vi "Convert Sample Rate MHz to and from Enum.vi"(10 "Sample Frequency enum in":T1=enum."100MHz", 11 "MHz in":u8) -> (2 "MHz out":u8, 3 "Sample Frequency enum out":T1=enum."200MHz (LT2 only)")   [LabVIEW 2026, in "MicroPulse_Driver.lvlib"]
uses:
  MicroPulse_Driver.lvlib
  Data/Datatypes/MP - sample frequency.ctl
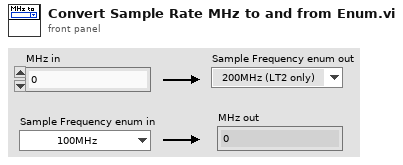
[diagram p1: front panel]
types:
  T1 = typedef "MicroPulse_Driver.lvlib/MP - sample frequency.ctl" = enum16{"Use Default", "200MHz (LT2 only)", "100MHz", "50MHz", "25MHz", "10MHz"}
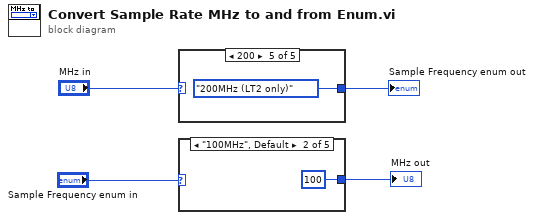
[diagram p0: block diagram]
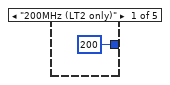
[diagram p2: hidden frame]
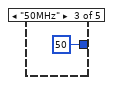
[diagram p3: hidden frame]
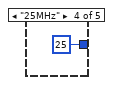
[diagram p4: hidden frame]
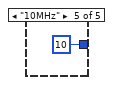
[diagram p5: hidden frame]
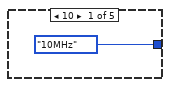
[diagram p6: hidden frame]
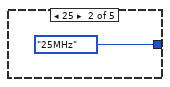
[diagram p7: hidden frame]
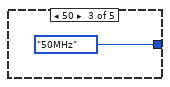
[diagram p8: hidden frame]
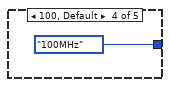
[diagram p9: hidden frame]
diagram:
  n1 = case shown="200" "MHz in" {
    tunnel: [MP_-_sample_frequency."10MHz" ("Sample Frequency") MP_-_sample_frequency."25MHz" ("Sample Frequency") MP_-_sample_frequency."50MHz" ("Sample Frequency") MP_-_sample_frequency."100MHz" ("Sample Frequency") MP_-_sample_frequency."200MHz (LT2 only)" ("Sample Frequency")] -> w4
    frame 10 {
    }
    frame 25 {
    }
    frame 50 {
    }
    frame 100, Default {
    }
    frame 200 {
    }
  }
  "Sample Frequency enum out" <- w4
  n2 = case shown="\"100MHz\", Default" "Sample Frequency enum in" {
    tunnel: [u8 200 ("MHz out") u8 100 ("MHz out") u8 50 ("MHz out") u8 25 ("MHz out") u8 10 ("MHz out")] -> w1
    frame "200MHz (LT2 only)" {
    }
    frame "100MHz", Default {
    }
    frame "50MHz" {
    }
    frame "25MHz" {
    }
    frame "10MHz" {
    }
  }
  "MHz out" <- w1
